vi "SmartMotor_single motor convert motion params v2.vi"(7 "Cnts ScaleFactors":T1, 8 "error in (no error)":errorcluster, 11 "motion params":T2) -> (0 "error out":errorcluster, 1 "accelCmd":string="ADT=0", 2 "velCmd":string="VT=0", 3 "posCmd":string="PT=0")   [LabVIEW 2020]
doc: "Developed by: Kevin Thompson\nThompson Engineering\nthompson.engineering@comcast.net\n(510) 673-3614"
uses:
  TD MotionParams--cluster.ctl
  TD PositionType_enum.ctl
  TD Cnts ScaleFactors - [EU to Cnts].ctl
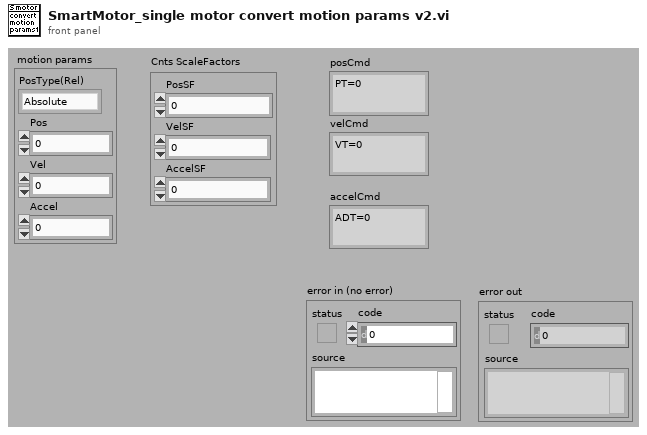
[diagram p1: front panel]
types:
  T1 = typedef "TD Cnts ScaleFactors - [EU to Cnts].ctl" = cluster{"PosSF":dbl, "VelSF":dbl, "AccelSF":dbl}
  T2 = typedef "TD MotionParams--cluster.ctl" = cluster{"PosType(Rel)":T3, "Pos":dbl, "Vel":dbl, "Accel":dbl}
  T3 = typedef "TD PositionType_enum.ctl" = enum16{"Absolute", "Relative"}
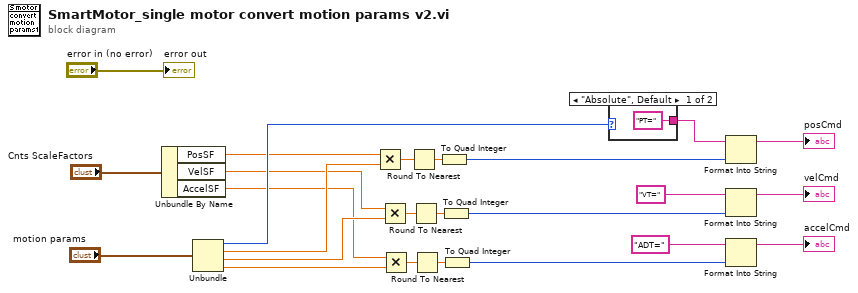
[diagram p0: block diagram]
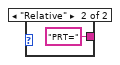
[diagram p2: hidden frame]
diagram:
  n1 = Unbundle By Name("Cnts ScaleFactors") -> ("PosSF"=w4:dbl, "VelSF"=w3:dbl, "AccelSF"=w2:dbl)
  n2 = Unbundle("motion params") -> ("PosType(Rel)"=w13:T3, "Pos"=w12:dbl, "Vel"=w11:dbl, "Accel"=w10:dbl)
  n3 = Multiply(x=w4, y=w12) -> (x*y=w15:dbl)
  n4 = Multiply(x=w3, y=w11) -> (x*y=w25:dbl)
  n5 = Multiply(x=w2, y=w10) -> (x*y=w22:dbl)
  n6 = Round To Nearest(number=w15) -> (nearest integer value=w14:dbl)
  n7 = Round To Nearest(number=w25) -> (nearest integer value=w24:dbl)
  n8 = Round To Nearest(number=w22) -> (nearest integer value=w23:dbl)
  n9 = To Quad Integer(1:w14) -> (0:w21:i64)
  n10 = To Quad Integer(1:w24) -> (0:w20:i64)
  n11 = To Quad Integer(1:w23) -> (0:w19:i64)
  n12 = case shown="\"Absolute\", Default" w13 {
    tunnel: ["PT=" "PRT="] -> w6
    frame "Absolute", Default {
    }
    frame "Relative" {
    }
  }
  n13 = Format Into String(initial string=w6, w21) -> (resulting string=→"posCmd":string)  [unwired: 2 in, 1 out]
  n14 = Format Into String(initial string="VT=", w20) -> (resulting string=→"velCmd":string)  [unwired: 2 in, 1 out]
  n15 = Format Into String(initial string="ADT=", w19) -> (resulting string=→"accelCmd":string)  [unwired: 2 in, 1 out]
  "error out" <- "error in (no error)"
